vi "Wait Clock.vi"(8 "First Time?":bool, 11 "Target Time":dbl) -> (3 "Completed":bool)   [LabVIEW 2015]
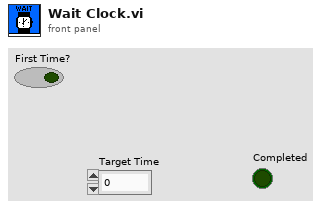
[diagram p1: front panel]
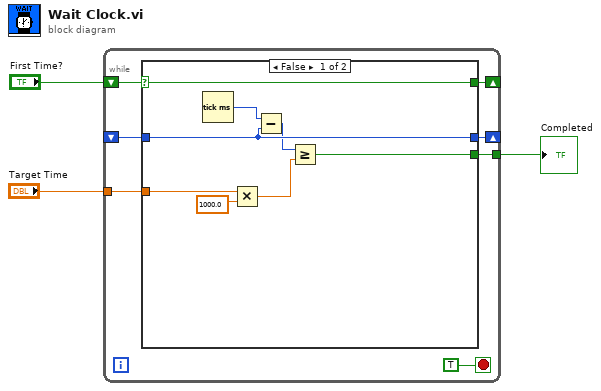
[diagram p0: block diagram]
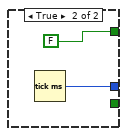
[diagram p2: hidden frame]
diagram:
  n1 = while {
    shift-right: [w10] -> _
    shift-left: _ -> [w9]
    tunnel: "Target Time" -> [w8]
    tunnel: [w7] -> w2
    shift-right: [w5] -> _
    shift-left: "First Time?" -> [w6]
    stop <- TRUE stop-if-true
    n2 = case shown="False" w6 {
      selector: w6 -> [w14 _]
      tunnel: [w17 w20] -> w10
      tunnel: w9 -> [w17 _]
      tunnel: w8 -> [w12 _]
      tunnel: [w15 _] -> w7
      tunnel: [w14 FALSE] -> w5
      frame False {
        n3 = Tick Count (ms)() -> (millisecond timer value=w18:u32)
        n4 = Multiply(x=w12, y=1000.0) -> (x*y=w13:dbl)
        n5 = Subtract(x=w18, y=w17) -> (x-y=w16:u32)
        n6 = Greater Or Equal?(x=w16, y=w13) -> (x >= y?=w15:bool)
      }
      frame True {
        n7 = Tick Count (ms)() -> (millisecond timer value=w20:u32)
      }
    }
  }
  "Completed" <- w2
